vi "XIPIN_Spartan-6_FPGA_GTP_Transceiver_Wizard_1_11.vi"   [LabVIEW 2017]
doc: "Use the Spartan-6 FPGA GTP Transceiver Wizard to configure one or more Spartan-6 FPGA GTPA1 transceivers. Start from scratch, or use an industry standard template. The Wizard generates a custom wrapper for the tranceivers you've selected. In addition, it produces an example design, testbench, and scripts to observe the transceivers operating under simulation and in hardware.\n------------------------------------\n<b>Need License</b> : No"
uses:
  <vilib>/rvi/XilinxIP/XIPIN_XNode/niFpgaXIPIN.xnode
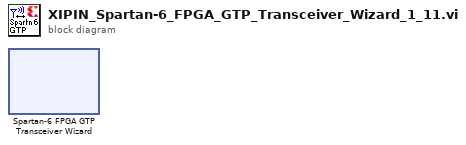
[diagram p0: block diagram]
diagram:
  n1 = xnode ("Spartan-6 FPGA GTP Transceiver Wizard")() -> ()
